vi "_Run Cycle.vi"(3 "Init (F)":bool, 4 "Update":bool) -> (1 "Finish Run?":bool)   [LabVIEW 2012]
uses:
  Instance           9 18Saved   _Run Cycle .vi
  <vilib>/rvi/DataTransferAndStorage/Container/Common/niFpgaContainerGetUniqueNameForEmu.vi
  <vilib>/rvi/Memory/Memory_Emulation/niFpgaMemoryEmulationCacheClearOnFirstRun.vi
  <vilib>/rvi/Memory/Memory_Emulation/nirvimemoryEmulationManagerCache_MakeExclusive.vi
  <vilib>/rvi/Memory/Memory_Emulation/niFpgaMemoryEmulationValidateCache.vi
  <vilib>/rvi/Memory/Memory_Emulation/nirvimemoryEmulationManagerCache_ReleaseExclusive.vi
  <vilib>/rvi/Memory/Memory_Emulation/nirvimemoryEmulationManagerCache_InsertValue.vi
  <vilib>/Utility/error.llb/Clear Errors.vi
  <vilib>/rvi/Memory/Memory_Emulation/nirvimemoryEmulationManagerCache_GetValue.vi
  <vilib>/rvi/Emulation/niFpgaSctlEmulationGetInTimedLoop.vi
  <vilib>/rvi/Memory/Memory_Emulation/nirvimemoryEmulationManagerCache_SetValue.vi
  <vilib>/rvi/Emulation/niFpgaSctlEmulationResourceMgr.vi
  <vilib>/rvi/DataTransferAndStorage/Container/XNode/niFpgaContainer.xnode
  <vilib>/rvi/Memory/Memory_Emulation/nirvimemoryEmulation.vi
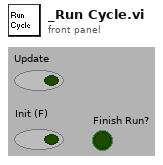
[diagram p1: front panel]
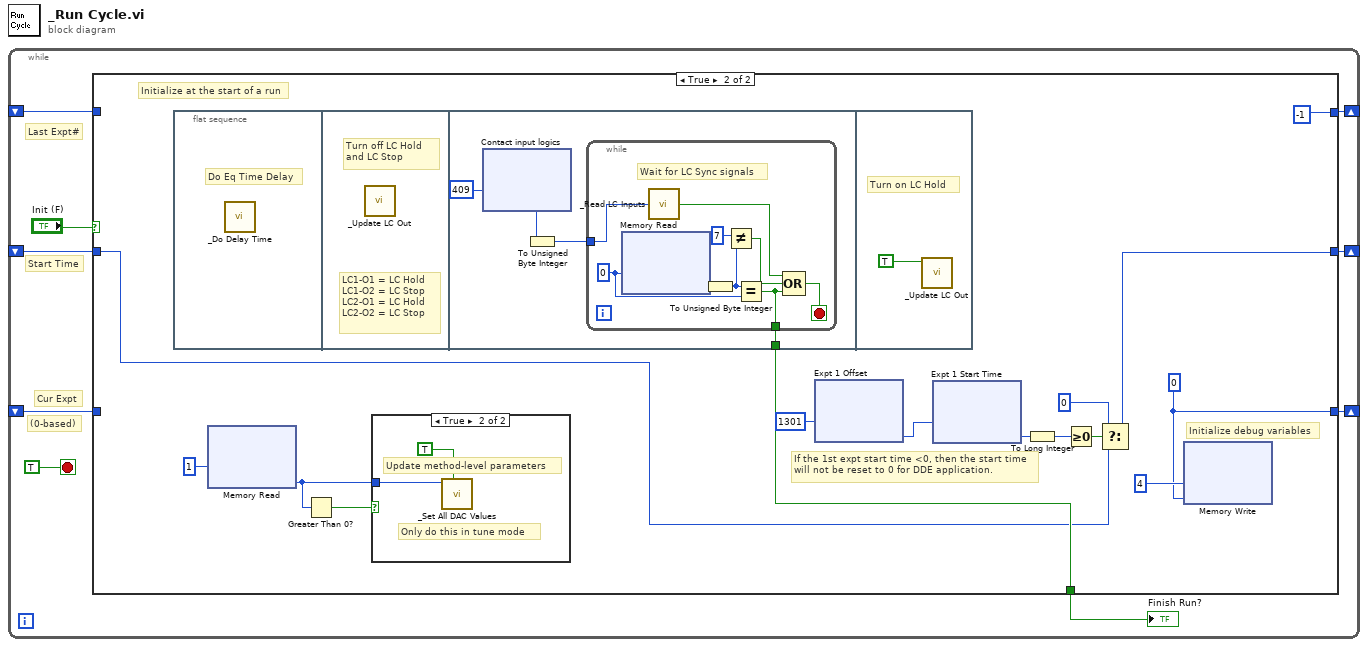
[diagram p0: block diagram]
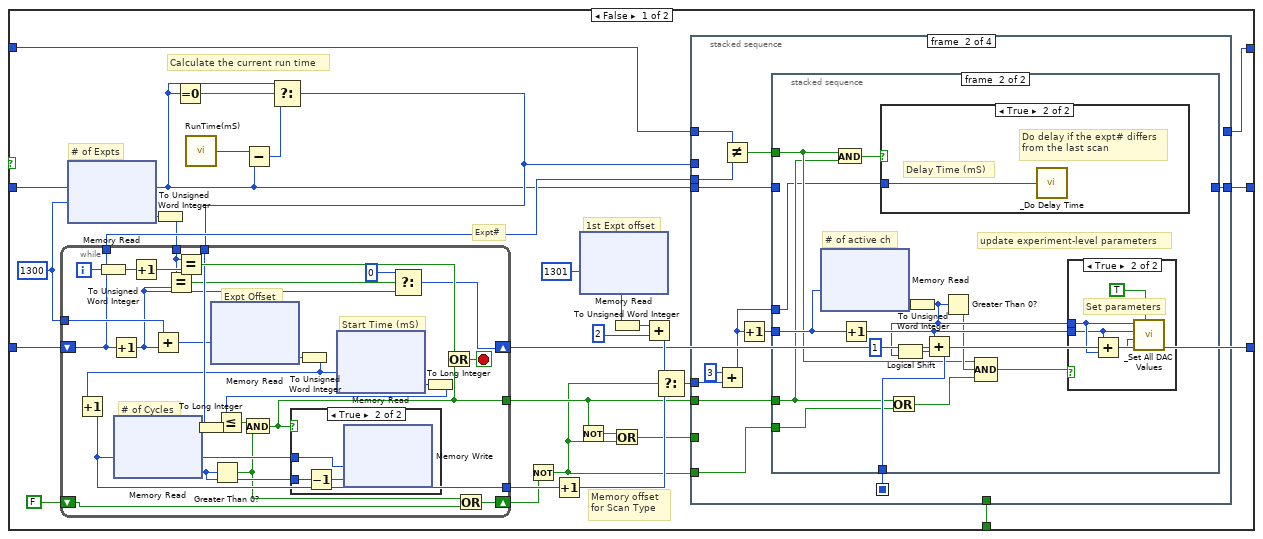
[diagram p2: hidden frame]
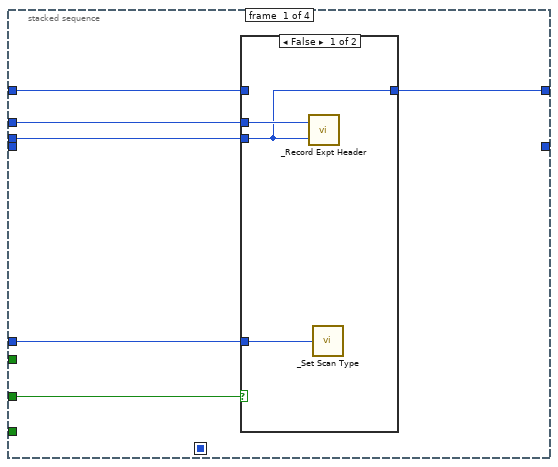
[diagram p3: hidden frame]
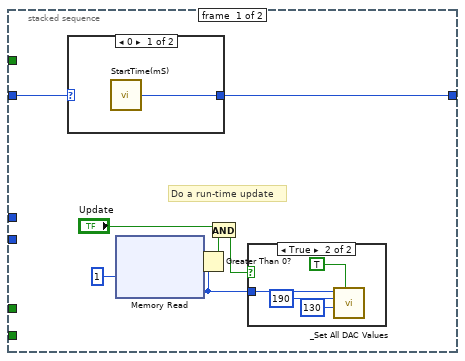
[diagram p5: hidden frame]
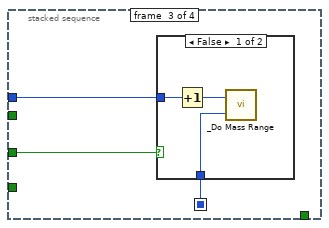
[diagram p10: hidden frame]
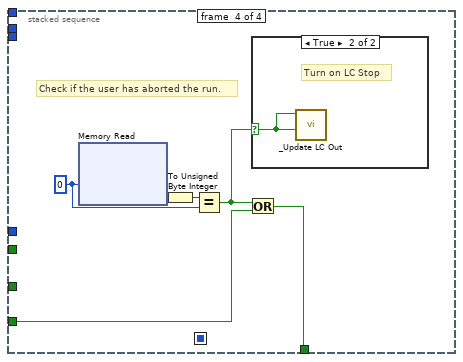
[diagram p12: hidden frame]
diagram:
  n1 = while {
    shift-right: [w8] -> _
    shift-left: _ -> [w7]
    shift-right: [w5] -> _
    shift-left: _ -> [w4]
    shift-right: [w2] -> _
    shift-left: _ -> [w1]
    stop <- TRUE stop-if-true
    # "Last Expt#"
    # "(0-based)"
    # "Cur Expt"
    # "Start Time"
    n2 = case shown="True" "Init (F)" {
      tunnel: [w13 w137] -> w8
      tunnel: w7 -> [w14 w138]
      tunnel: [w25 w140] -> w5
      tunnel: w4 -> [w28 _]
      tunnel: [w26 w148] -> w3
      tunnel: [w10 i16 -1 ("Data")] -> w2
      tunnel: w1 -> [w11 _]
      frame False {
        w37 = u16 1300 ("Address")
        # "Calculate the current run time"
        # "Memory offset\nfor Scan Type"
        # "1st Expt offset"
        # "# of Expts"
        # "Expt#"
        n3 = xnode ("Memory Read")("Address"=w37) -> ("Data"=w36:u32)  [unwired: 1 in, 1 out]
        n4 = To Unsigned Word Integer(number=w36) -> (unsigned 16bit integer=w12:u16)
        n5 = Equal To 0?(x=w14) -> (x = 0?=w17:bool)
        n6 = call "RunTime(mS)"() -> ("Tick Count(mSec)"=w27:u32)
        n7 = Subtract(x=w27, y=w14) -> (x-y=w16:u32)
        n8 = Select(t=w14, s=w17, f=w16) -> (s? t:f=w15:u32)
        n9 = while {
          tunnel: w15 -> [w129]
          shift-right: [w119] -> w25
          shift-left: w28 -> [w114]
          tunnel: [w116] -> w38
          tunnel: w12 -> [w122]
          tunnel: w37 -> [w125]
          tunnel: [w114] -> w24
          shift-right: [w113] -> w22
          shift-left: FALSE -> [w112]
          tunnel: [w110] -> w20
          i -> [w128]
          stop <- w131 stop-if-true
          # "# of Cycles"
          # "Start Time (mS)"
          # "Expt Offset"
          n10 = To Unsigned Word Integer(number=w128) -> (unsigned 16bit integer=w124:u16)
          n11 = Increment(x=w114) -> (x+1=w115:u16)
          n12 = Increment(x=w124) -> (x+1=w123:u16)
          n13 = Add(x=w125, y=w115) -> (x+y=w127:u16)
          n14 = Equal?(x=w122, y=w115) -> (x = y?=w121:bool)
          n15 = Equal?(x=w122, y=w123) -> (x = y?=w130:bool)
          n16 = To Long Integer(number=w129) -> (32bit integer=w107:i32)
          n17 = xnode ("Memory Read")("Address"=w127) -> ("Data"=w126:u32)  [unwired: 1 in, 1 out]
          n18 = To Unsigned Word Integer(number=w126) -> (unsigned 16bit integer=w118:u16)
          n19 = Increment(x=w118) -> (x+1=w116:u16)
          n20 = xnode ("Memory Read")("Address"=w116) -> ("Data"=w117:u32)  [unwired: 1 in, 1 out]
          n21 = Greater Than 0?(x=w117) -> (x > 0?=w111:bool)
          n22 = xnode ("Memory Read")("Address"=w118) -> ("Data"=w109:u32)  [unwired: 1 in, 1 out]
          n23 = Select(t=u16 0, s=w121, f=w115) -> (s? t:f=w119:u16)
          n24 = To Long Integer(number=w109) -> (32bit integer=w108:i32)
          n25 = Less Or Equal?(x=w108, y=w107) -> (x <= y?=w132:bool)
          n26 = And(x=w132, y=w111) -> (x .and. y?=w110:bool)
          n27 = case shown="True" w110 {
            tunnel: w117 -> [_ w134]
            tunnel: w116 -> [_ w135]
            frame False {
            }
            frame True {
              n28 = Decrement(x=w134) -> (x-1=w133:u32)
              n29 = xnode ("Memory Write")("Address"=w135, "Data"=w133) -> ()  [unwired: 1 in, 1 out]
            }
          }
          n30 = Or(x=w130, y=w110) -> (x .or. y?=w131:bool)
          n31 = Or(x=w111, y=w112) -> (x .or. y?=w113:bool)
        }
        n32 = Not(x=w22) -> (.not. x?=w19:bool)
        n33 = Increment(x=w38) -> (x+1=w29:u16)
        n34 = Not(x=w20) -> (.not. x?=w21:bool)
        n35 = xnode ("Memory Read")("Address"=u16 1301) -> ("Data"=w33:u32)  [unwired: 1 in, 1 out]
        n36 = To Unsigned Word Integer(number=w33) -> (unsigned 16bit integer=w32:u16)
        n37 = Or(x=w21, y=w19) -> (x .or. y?=w18:bool)
        n38 = Add(x=w32, y=u8 2) -> (x+y=w31:u16)
        n39 = Select(t=w31, s=w19, f=w29) -> (s? t:f=w30:u16)
        n40 = stacked-sequence {
          seq-local: [_ w59 _ _] -> [_ _ w96 _]
          tunnel: w15 -> [w41 _ _ _]
          tunnel: w24 -> [w44 w50 _ _]
          tunnel: w30 -> [w42 w54 w95 _]
          tunnel: w19 -> [_ w55 _ w102]
          tunnel: [_ _ _ w101] -> w26
          tunnel: w20 -> [_ w56 _ _]
          tunnel: w18 -> [w43 _ w94 _]
          tunnel: w14 -> [_ w53 _ _]
          tunnel: [_ w52 _ _] -> w13
          tunnel: w11 -> [w40 w51 _ _]
          tunnel: [w39 _ _ _] -> w10
          frame #0 {
            n41 = case shown="False" w43 {
              tunnel: w41 -> [w46 _]
              tunnel: w44 -> [w45 _]
              tunnel: w42 -> [w47 _]
              tunnel: w40 -> [_ w48]
              tunnel: [w45 w48] -> w39
              frame False {
                n42 = call "_Record Expt Header.vi"("Expt/Cycle#"=w45, "Run Time (mS)"=w46) -> ()  [unwired: 1 out]
                n43 = call "_Set Scan Type.vi"("ScanType Offset"=w47) -> ()
              }
              frame True {
                # "Pause period or finish run."
              }
            }
          }
          frame #1 {
            n44 = Add(x=u8 3, y=w54) -> (x+y=w57:u16)
            n45 = Not Equal?(x=w51, y=w50) -> (x != y?=w49:bool)
            n46 = Increment(x=w57) -> (x+1=w60:u16)
            n47 = stacked-sequence {
              tunnel: w60 -> [_ w88]
              tunnel: [_ w87] -> w59
              tunnel: w57 -> [_ w74]
              tunnel: w56 -> [_ w76]
              tunnel: w55 -> [_ w86]
              tunnel: w53 -> [w67 _]
              tunnel: [w66 _] -> w52
              tunnel: w49 -> [_ w77]
              frame #0 {
                # "Do a run-time update"
                n48 = case shown="0" w67 {
                  selector: w67 -> [_ w73]
                  tunnel: [w72 w73] -> w66
                  frame 0 {
                    n49 = call "StartTime(mS)"() -> ("Tick Count(mSec)"=w72:u32)
                  }
                  frame 1, Default {
                  }
                }
                n50 = xnode ("Memory Read")("Address"=u8 1) -> ("Data"=w62:u32)  [unwired: 1 in, 1 out]
                n51 = Greater Than 0?(x=w62) -> (x > 0?=w64:bool)
                n52 = And(x="Update", y=w64) -> (x .and. y?=w63:bool)
                n53 = case shown="True" w63 {
                  tunnel: w62 -> [_ w69]
                  frame False {
                  }
                  frame True {
                    n54 = call "_Set All DAC Values.vi"("Record Values (F)"=TRUE, "DAC Value Offset (70)"=u16 130 ("DAC Value Offset (110)"), "Channel ID Offset (10)"=u16 190, "# of Active Channels"=w69) -> ()  [unwired: 5 in]
                  }
                }
              }
              frame #1 {
                # "update experiment-level parameters"
                # "# of active ch"
                n55 = xnode ("Memory Read")("Address"=w88) -> ("Data"=w82:u32)  [unwired: 1 in, 1 out]
                n56 = And(x=w77, y=w76) -> (x .and. y?=w75:bool)
                n57 = Increment(x=w88) -> (x+1=w83:u16)
                n58 = case shown="True" w75 {
                  tunnel: w74 -> [_ w89]
                  frame False {
                    # "No Pause for Subsequent Cycles\nor single experiment method"
                  }
                  frame True {
                    # "Delay Time (mS)"
                    # "Do delay if the expt# differs\nfrom the last scan"
                    n59 = call "_Do Delay Time.vi"("DelayTime Address"=w89) -> ()
                  }
                }
                n60 = Or(x=w76, y=w86) -> (x .or. y?=w78:bool)
                n61 = To Unsigned Word Integer(number=w82) -> (unsigned 16bit integer=w81:u16)
                n62 = Logical Shift(y=u8 1, x=w81) -> (x << y=w84:u16)
                n63 = Add(x=w83, y=w84) -> (x+y=w87:u16)
                n64 = Greater Than 0?(x=w81) -> (x > 0?=w80:bool)
                n65 = Compound Arithmetic op=AND(w77, w80, w78) -> (w79:bool)
                n66 = case shown="True" w79 {
                  tunnel: w81 -> [_ w92]
                  tunnel: w83 -> [_ w91]
                  frame False {
                    # "Pause Period"
                  }
                  frame True {
                    # "Set parameters"
                    n67 = Add(x=w91, y=w92) -> (x+y=w93:u16)
                    n68 = call "_Set All DAC Values.vi"("Record Values (F)"=TRUE, "DAC Value Offset (70)"=w93, "Channel ID Offset (10)"=w91, "# of Active Channels"=w92) -> ()  [unwired: 5 in]
                  }
                }
              }
            }
          }
          frame #2 {
            n69 = case shown="False" w94 {
              tunnel: w96 -> [w99 _]
              tunnel: w95 -> [w98 _]
              frame False {
                n70 = Increment(x=w98) -> (x+1=w97:u16)
                n71 = call "_Do Mass Range.vi"("# of MR Offset"=w99, "Pause Time Offset"=w97) -> ()  [unwired: 2 out]
              }
              frame True {
                # "Pause Period\nor Finish Run"
              }
            }
          }
          frame #3 {
            w105 = u8 0 ("Address")
            # "Check if the user has aborted the run."
            n72 = xnode ("Memory Read")("Address"=w105) -> ("Data"=w103:u32)  [unwired: 1 in, 1 out]
            n73 = To Unsigned Byte Integer(number=w103) -> (unsigned 8bit integer=w104:u8)
            n74 = Equal?(x=w104, y=w105) -> (x = y?=w100:bool)
            n75 = Or(x=w100, y=w102) -> (x .or. y?=w101:bool)
            n76 = case shown="True" w100 {
              selector: w100 -> [_ w106]
              frame False {
              }
              frame True {
                # "Turn on LC Stop"
                n77 = call "_Update LC Out.vi"("LC Stop"=w106, "LC Hold"=w106) -> ()  [unwired: 6 out]
              }
            }
          }
        }
      }
      frame True {
        w140 = u16 0 ("Data")
        # "If the 1st expt start time <0, then the start time\nwill not be reset to 0 for DDE application."
        # "Initialize debug variables"
        # "Initialize at the start of a run"
        n78 = flat-sequence {
          tunnel: [w156] -> w148
          frame #0 {
            # "Do Eq Time Delay"
            n79 = call "_Do Delay Time.vi"() -> ()  [unwired: 1 in]
          }
          frame #1 {
            # "Turn off LC Hold \nand LC Stop"
            # "LC1-O1 = LC Hold\nLC1-O2 = LC Stop\nLC2-O1 = LC Hold\nLC2-O2 = LC Stop"
            n80 = call "_Update LC Out.vi"() -> ()  [unwired: 2 in, 6 out]
          }
          frame #2 {
            n81 = xnode "Contact input logics"("Address"=u16 409) -> ("Data"=w154:u32)  [unwired: 1 in, 1 out]
            n82 = To Unsigned Byte Integer(number=w154) -> (unsigned 8bit integer=w153:u8)
            n83 = while {
              tunnel: [w162] -> w156
              tunnel: w153 -> [w157]
              stop <- w163 stop-if-true
              w164 = u8 0 ("Address")
              # "Wait for LC Sync signals"
              n84 = xnode ("Memory Read")("Address"=w164) -> ("Data"=w165:u32)  [unwired: 1 in, 1 out]
              n85 = call "_Read LC Inputs.vi"("LogicOption"=w157) -> ("LC Input Detected"=w158:bool)
              n86 = To Unsigned Byte Integer(number=w165) -> (unsigned 8bit integer=w161:u8)
              n87 = Not Equal?(x=u8 7, y=w161) -> (x != y?=w159:bool)
              n88 = Equal?(x=w161, y=w164) -> (x = y?=w162:bool)
              n89 = Compound Arithmetic op=OR(w158, w159, w162) -> (w163:bool)
            }
          }
          frame #3 {
            # "Turn on LC Hold"
            n90 = call "_Update LC Out.vi"("LC Hold"=TRUE ("Port5/DIO5")) -> ()  [unwired: 1 in, 6 out]
          }
        }
        n91 = xnode ("Memory Read")("Address"=u8 1) -> ("Data"=w147:u32)  [unwired: 1 in, 1 out]
        n92 = Greater Than 0?(x=w147) -> (x > 0?=w146:bool)
        n93 = case shown="True" w146 {
          tunnel: w147 -> [_ w152]
          frame False {
          }
          frame True {
            # "Update method-level parameters"
            # "Only do this in tune mode"
            n94 = call "_Set All DAC Values.vi"("Record Values (F)"=TRUE, "# of Active Channels"=w152) -> ()  [unwired: 7 in]
          }
        }
        n95 = xnode "Expt 1 Offset"("Address"=u16 1301) -> ("Data"=w144:u32)  [unwired: 1 in, 1 out]
        n96 = xnode "Expt 1 Start Time"("Address"=w144) -> ("Data"=w143:u32)  [unwired: 1 in, 1 out]
        n97 = To Long Integer(number=w143) -> (32bit integer=w142:i32)
        n98 = Greater Or Equal To 0?(x=w142) -> (x >= 0?=w141:bool)
        n99 = Select(t=u32 0 ("Tick Count(mSec)"), s=w141, f=w138) -> (s? t:f=w137:u32)
        n100 = xnode ("Memory Write")("Address"=u8 4, "Data"=w140) -> ()  [unwired: 1 in, 1 out]
      }
    }
    "Finish Run?" <- w3
  }
